vi "Vertical Slider.vi"() -> ()   [LabVIEW 2013]
panel:
  in  "stop":bool
  in  "Slide":dbl(slide) min=0.0 max=100.0 step=1.0 scale=0.0..100.0 scale format="%#_3g"
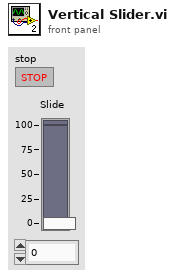
[diagram p1: front panel]
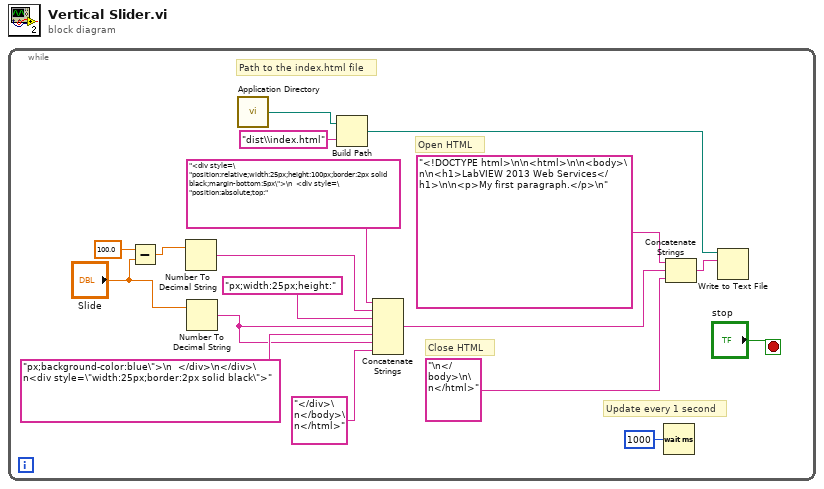
[diagram p0: block diagram]
diagram:
  n1 = while {
    stop <- "stop" stop-if-true
    # "Open HTML"
    # "Close HTML"
    # "Update every 1 second"
    # "Path to the index.html file"
    n2 = Subtract(x=100.0, y="Slide") -> (x-y=w5:dbl)
    n3 = Number To Decimal String(number=w5) -> (decimal integer string=w7:string)  [unwired: 1 in]
    n4 = Number To Decimal String(number="Slide") -> (decimal integer string=w2:string)  [unwired: 1 in]
    n5 = call <vilib>:"Application Directory.vi"() -> ("Application Directory"=w17:path)
    n6 = Build Path(base path=w17, name or relative path="dist\\index.html") -> (appended path=w11:path)
    n7 = Concatenate Strings("<div style=\"position:relative;width:25px;height:100px;border:2px solid black;margin-bottom:5px\">\n  <div style=\"position:absolute;top:", w7, "px;width:25px;height:" ("string"), w2, "px;background-color:blue\">\n  </div>\n</div>\n<div style=\"width:25px;border:2px solid black\">" ("string"), w2, "</div>\n</body>\n</html>") -> (w13:string)
    n8 = Wait (ms)(milliseconds to wait=u32 1000) -> ()  [unwired: 1 out]
    n9 = Concatenate Strings("<!DOCTYPE html>\n\n<html>\n\n<body>\n\n<h1>LabVIEW 2013 Web Services</h1>\n\n<p>My first paragraph.</p>\n", w13, "\n</body>\n\n</html>") -> (w12:string)
    n10 = Write to Text File(file (use dialog)=w11, text=w12) -> ()  [unwired: 2 in, 3 out]
  }
